vi "Delete Bucket Website Configuration.vi"(8 "error in (no error)":errorcluster, 9 "Bucket":string) -> (0 "error out":errorcluster)   [LabVIEW 2011, in "LV Interface for Amazon S3.lvlib"]
doc: "<B>Removes</B> the <B>website configuration</B> for a bucket. This operation <B>requires</B> the <B>S3:DeleteBucketWebsite permission</B>. By default, only the bucket owner can delete the website configuration attached to a bucket. Bucket <B>owners can grant</B> other <B>users permission to delete the website configuration</B> by writing a bucket policy <B>granting them the S3:DeleteBucketWebsite permission</B>."
uses:
  LV Interface for Amazon S3.lvlib
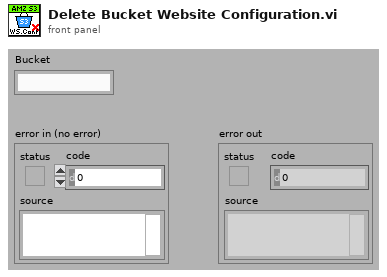
[diagram p1: front panel]
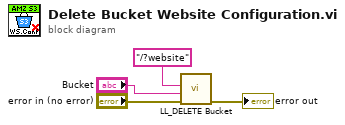
[diagram p0: block diagram]
diagram:
  n1 = call "LL_DELETE Bucket.vi"("error in (no error)"="error in (no error)", "Bucket"="Bucket", "Path and query string"="/?website") -> ("error out"=→"error out":errorcluster)  [unwired: 7 in, 1 out]
